vi "Move-Turn-Gear.vi"(6 "toGear":dbl, 8 "error in (no error)":errorcluster, 9 "gearDistance":dbl, 10 "Position":string, 11 "PID gains":T1={"proportional gain (Kc)"=0.085, "integral time (Ti, min)"=0.0, "derivative time (Td, min)"=0.0}) -> (0 "error out":errorcluster)   [LabVIEW 2016]
panel:
  out "PID gains 2":T1(graph)
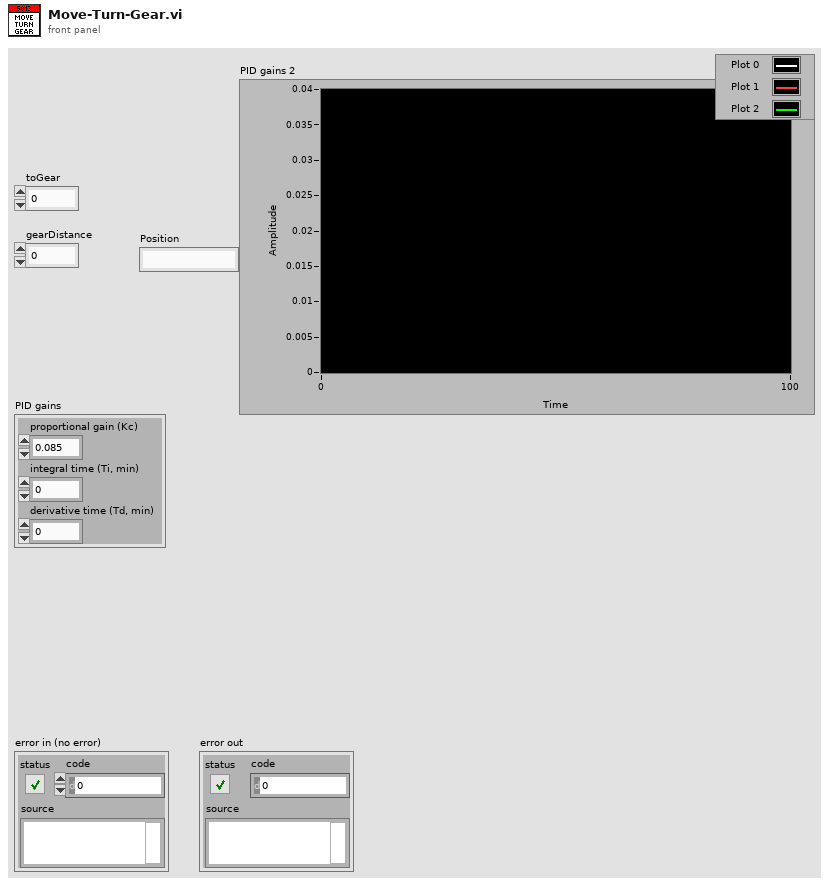
[diagram p1: front panel]
types:
  T1 = cluster{"proportional gain (Kc)":dbl, "integral time (Ti, min)":dbl, "derivative time (Td, min)":dbl}
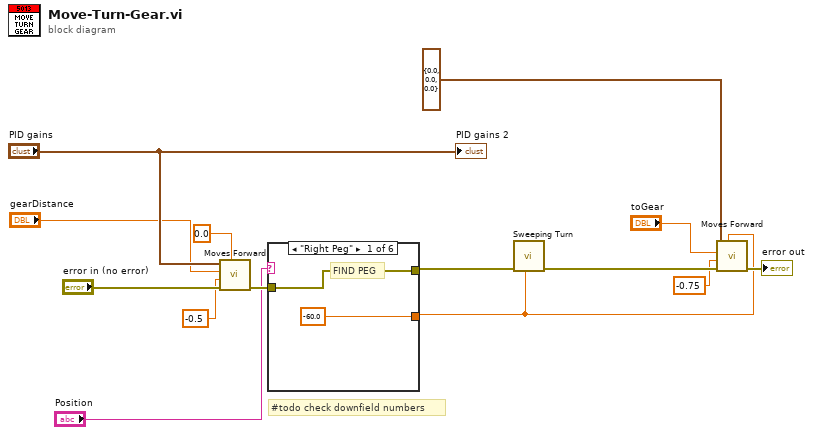
[diagram p0: block diagram]
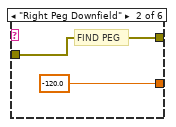
[diagram p2: hidden frame]
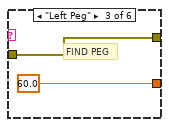
[diagram p3: hidden frame]
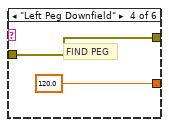
[diagram p4: hidden frame]
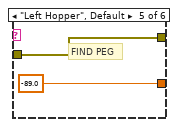
[diagram p5: hidden frame]
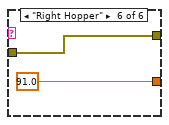
[diagram p6: hidden frame]
diagram:
  # "#todo check downfield numbers"
  n1 = call "Moves Forward.vi"("yaw setpoint"=0.0, "error in (no error)"="error in (no error)", "Speed"=-0.5, "forwardDistance"="gearDistance", "PID gains"="PID gains") -> ("error out"=w9:errorcluster)  [unwired: 4 in, 2 out]
  n2 = case shown="\"Right Peg\"" "Position" {
    tunnel: w9 -> [w15 w17 w19 w21 w23 w25]
    tunnel: [w15 w17 w19 w21 w23 w25] -> w10
    tunnel: [-60.0 ("upper limit right") -120.0 ("upper limit right") 60.0 ("upper limit left") 120.0 ("upper limit left") -89.0 ("upper limit left") 91.0 ("upper limit left")] -> w2
    frame "Right Peg" {
      # "FIND PEG"
    }
    frame "Right Peg Downfield" {
      # "FIND PEG"
    }
    frame "Left Peg" {
      # "FIND PEG"
    }
    frame "Left Peg Downfield" {
      # "FIND PEG"
    }
    frame "Left Hopper", Default {
      # "FIND PEG"
    }
    frame "Right Hopper" {
    }
  }
  n3 = call "Sweeping Turn.vi"("upper angle limit"=w2, "error in"=w10) -> ("error out"=w11:errorcluster)  [unwired: 9 in]
  n4 = call "Moves Forward.vi"("yaw setpoint"=w2, "error in (no error)"=w11, "Speed"=-0.75, "forwardDistance"="toGear", "PID gains"=T1 {"proportional gain (Kc)"=0.0, "integral time (Ti, min)"=0.0, "derivative time (Td, min)"=0.0}) -> ("error out"=→"error out":errorcluster)  [unwired: 4 in, 2 out]
  "PID gains 2" <- "PID gains"
